vi "BlurredRegistration.vi"(8 "error in":errorcluster, 9 "Gaussian blur parameters":T1={"large sigma"=20.0, "small sigma"=4.0, "equalize?"=FALSE}, 10 "roy":T2, 11 "rob":T2) -> (0 "error out":errorcluster, 1 "alignment quality":dbl, 2 "y displacement":dbl, 3 "x displacement":dbl)   [LabVIEW 2012]
uses:
  <vilib>/vision/Image Controls.llb/IMAQ Image.ctl
  Gaussian blur parameters.ctl
  <vilib>/vision/NI_Vision_Development_Module.lvlib
panel:
  out "gaussian roy":T2(plugin-control)
  out "gaussian rob":T2(plugin-control)
  out "gaussian cc":T2(plugin-control)
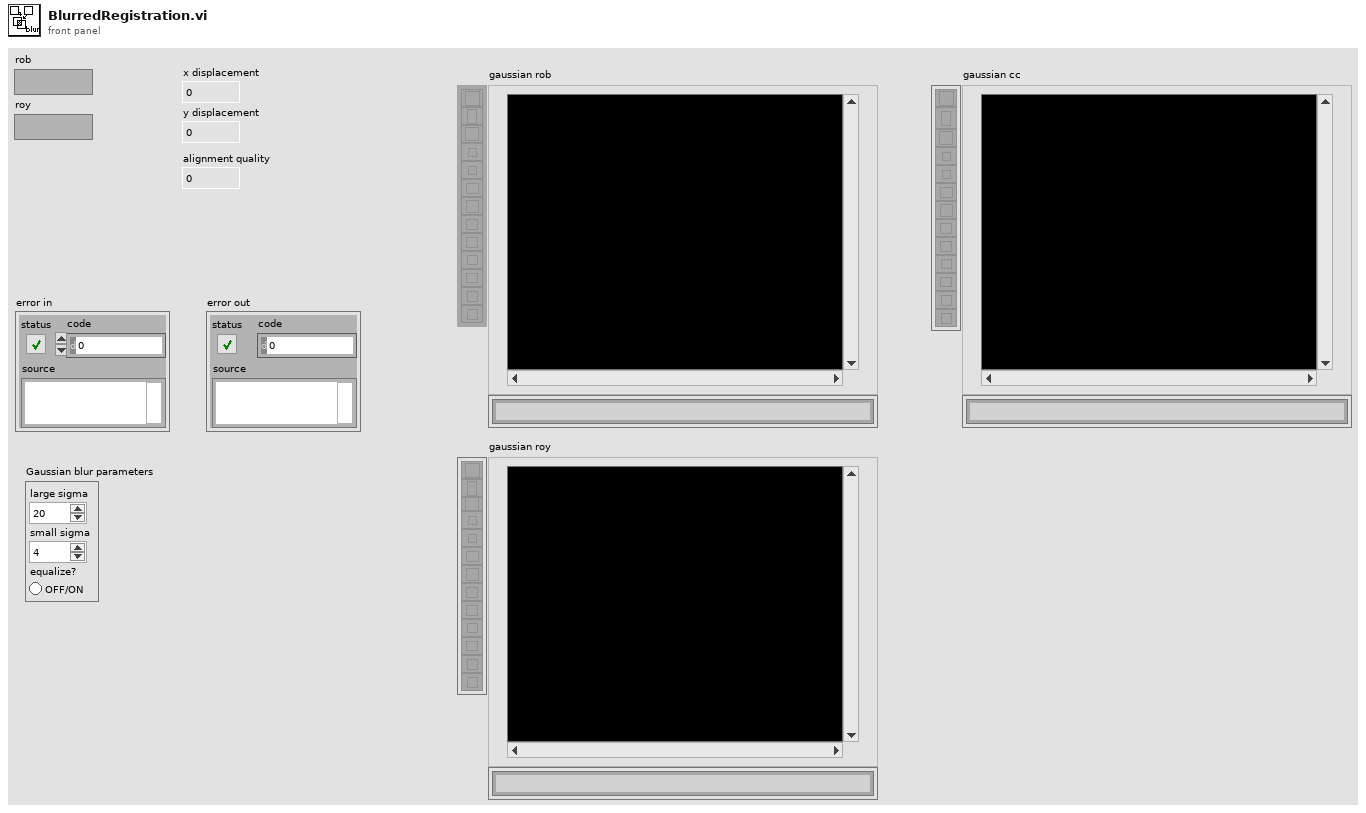
[diagram p1: front panel]
types:
  T1 = typedef "Gaussian blur parameters.ctl" = cluster{"large sigma":sgl, "small sigma":sgl, "equalize?":bool}
  T2 = typedef "IMAQ Image.ctl" = refnum<image>
  T3 = typedef "Image Type" = u32
  T4 = cluster{"histogram":u32[], "Minimal Value":sgl, "Maximal Value":sgl, "Starting Value":sgl, "Interval Width":sgl, "Mean Value":sgl, "Standard  Variation":sgl, "Area (pixels)":i32}
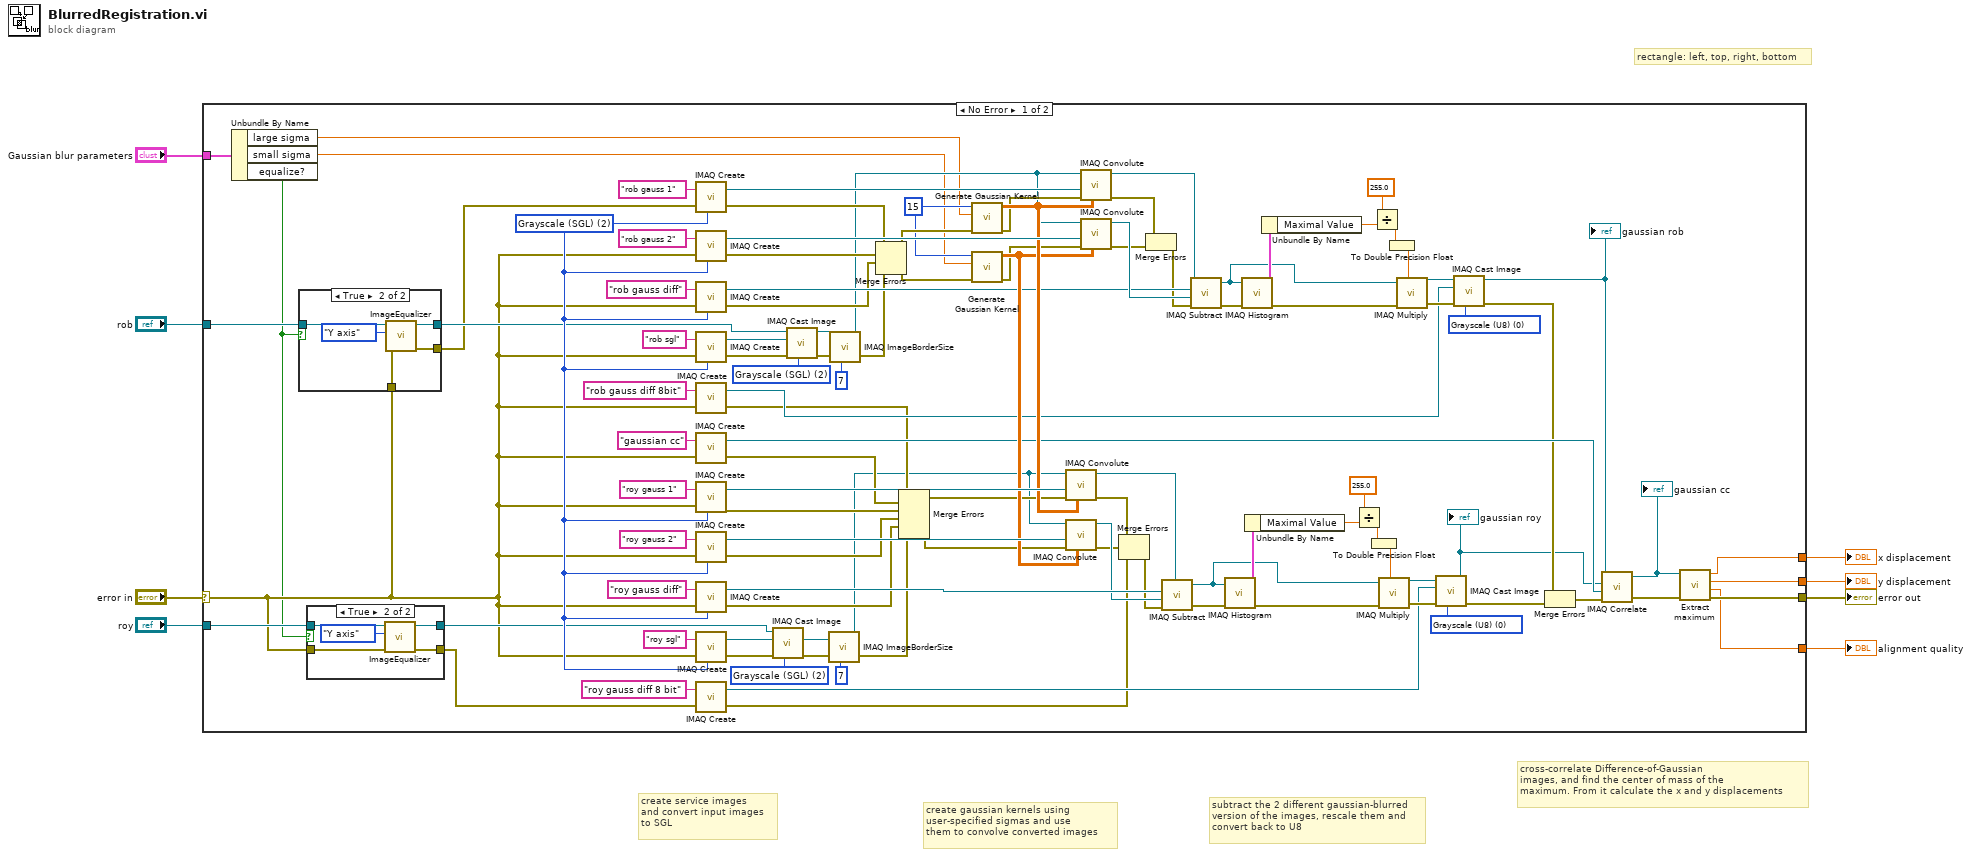
[diagram p0: block diagram]
diagram:
  # "rectangle: left, top, right, bottom"
  # "cross-correlate Difference-of-Gaussian\nimages, and find the center of mass of the \nmaximum. From it calculate the x and y displacements"
  # "subtract the 2 different gaussian-blurred\nversion of the images, rescale them and \nconvert back to U8"
  # "create gaussian kernels using\nuser-specified sigmas and use \nthem to convolve converted images"
  # "create service images\nand convert input images\nto SGL"
  n1 = case shown="No Error" "error in" {
    selector: "error in" -> [w21 w130]
    tunnel: [w17 w130] -> w7
    tunnel: "roy" -> [w23 _]
    tunnel: "rob" -> [w26 _]
    tunnel: [w15 _] -> w3
    tunnel: [w16 _] -> w2
    tunnel: [w14 _] -> w4
    tunnel: "Gaussian blur parameters" -> [w12 _]
    frame No Error {
      w35 = T3 2 items=["Grayscale (U8)", "Grayscale (I16)", "Grayscale (SGL)", "Complex (CSG)", "RGB (U32)", "HSL (U32)", "RGB (U64)", "Grayscale (U16)"] ("Image Type")
      w40 = T3 2 items=["Grayscale (U8)", "Grayscale (I16)", "Grayscale (SGL)", "Complex (CSG)", "RGB (U32)", "HSL (U32)", "RGB (U64)", "Grayscale (U16)"] ("Image Type")
      w55 = T3 0 items=["Grayscale (U8)", "Grayscale (I16)", "Grayscale (SGL)", "Complex (CSG)", "RGB (U32)", "HSL (U32)", "RGB (U64)", "Grayscale (U16)"] ("Image Type")
      w62 = T3 0 items=["Grayscale (U8)", "Grayscale (I16)", "Grayscale (SGL)", "Complex (CSG)", "RGB (U32)", "HSL (U32)", "RGB (U64)", "Grayscale (U16)"] ("Image Type")
      w73 = T3 2 items=["Grayscale (U8)", "Grayscale (I16)", "Grayscale (SGL)", "Complex (CSG)", "RGB (U32)", "HSL (U32)", "RGB (U64)", "Grayscale (U16)"] ("Image Type")
      w76 = 15 ("kernel size (odd number)")
      n2 = Unbundle By Name(w12) -> ("large sigma"=w11:sgl, "small sigma"=w10:sgl, "equalize?"=w9:bool)
      n3 = case shown="True" w9 {
        tunnel: w26 -> [w124 w129]
        tunnel: [w124 w128] -> w25
        tunnel: [w123 w126] -> w24
        tunnel: w21 -> [w123 w125]
        frame False {
        }
        frame True {
          n4 = call "ImageEqualizer.vi"("error in (no error)"=w125, "axis to equalize"=enum16{"X axis", "Y axis"}."Y axis", "Image in"=w129) -> ("error out"=w126:errorcluster, "Image out"=w128:T2)  [unwired: 7 in]
        }
      }
      n5 = case shown="True" w9 {
        tunnel: w23 -> [w117 w121]
        tunnel: [w117 w120] -> w22
        tunnel: w21 -> [w116 w119]
        tunnel: [w116 w118] -> w13
        frame False {
        }
        frame True {
          n6 = call "ImageEqualizer.vi"("error in (no error)"=w119, "axis to equalize"=enum16{"X axis", "Y axis"}."Y axis", "Image in"=w121) -> ("error out"=w118:errorcluster, "Image out"=w120:T2)  [unwired: 7 in]
        }
      }
      n7 = call "IMAQ Create"("Image Name"="rob gauss 1", "Image Type"=w73, "error in (no error)"=w24) -> ("New Image"=w104:T2, "error out"=w92:errorcluster)  [unwired: 2 in]
      n8 = call "IMAQ Create"("Image Name"="rob gauss 2", "Image Type"=w73, "error in (no error)"=w21) -> ("New Image"=w103:T2, "error out"=w91:errorcluster)  [unwired: 2 in]
      n9 = call "IMAQ Create"("Image Name"="rob gauss diff", "Image Type"=w73, "error in (no error)"=w21) -> ("New Image"=w96:T2, "error out"=w90:errorcluster)  [unwired: 2 in]
      n10 = call "IMAQ Create"("Image Name"="rob sgl", "Image Type"=w73, "error in (no error)"=w21) -> ("New Image"=w44:T2, "error out"=w43:errorcluster)  [unwired: 2 in]
      n11 = call "IMAQ Create"("Image Name"="rob gauss diff 8bit", "error in (no error)"=w21) -> ("New Image"=w63:T2, "error out"=w33:errorcluster)  [unwired: 3 in]
      n12 = call "IMAQ Create"("Image Name"="gaussian cc", "error in (no error)"=w21) -> ("New Image"=w70:T2, "error out"=w34:errorcluster)  [unwired: 3 in]
      n13 = call "IMAQ Create"("Image Name"="roy gauss 1", "Image Type"=w73, "error in (no error)"=w21) -> ("New Image"=w102:T2, "error out"=w82:errorcluster)  [unwired: 2 in]
      n14 = call "IMAQ Create"("Image Name"="roy gauss 2", "Image Type"=w73, "error in (no error)"=w21) -> ("New Image"=w101:T2, "error out"=w83:errorcluster)  [unwired: 2 in]
      n15 = call "IMAQ Create"("Image Name"="roy gauss diff", "Image Type"=w73, "error in (no error)"=w21) -> ("New Image"=w95:T2, "error out"=w81:errorcluster)  [unwired: 2 in]
      n16 = call "IMAQ Create"("Image Name"="roy sgl", "Image Type"=w73, "error in (no error)"=w21) -> ("New Image"=w39:T2, "error out"=w37:errorcluster)  [unwired: 2 in]
      n17 = call "IMAQ Create"("Image Name"="roy gauss diff 8 bit", "error in (no error)"=w13) -> ("New Image"=w53:T2, "error out"=w29:errorcluster)  [unwired: 3 in]
      n18 = call "IMAQ Cast Image"("Image Type"=w35, "error in (no error)"=w37, "Image Dst"=w39, "Image Src"=w22) -> ("error out"=w36:errorcluster, "Image Dst Out"=w38:T2)  [unwired: 6 in]
      n19 = call "IMAQ Cast Image"("Image Type"=w40, "error in (no error)"=w43, "Image Dst"=w44, "Image Src"=w25) -> ("error out"=w42:errorcluster, "Image Dst Out"=w41:T2)  [unwired: 6 in]
      n20 = call "IMAQ ImageBorderSize"("Image"=w38, "Image border size in"=7, "error in (no error)"=w36) -> ("Image Out"=w30:T2, "error out"=w31:errorcluster)  [unwired: 1 in, 1 out]
      n21 = call "IMAQ ImageBorderSize"("Image"=w41, "Image border size in"=7, "error in (no error)"=w42) -> ("Image Out"=w72:T2, "error out"=w32:errorcluster)  [unwired: 1 in, 1 out]
      n22 = Merge Errors(w92, w91, w90, w32) -> (w89:errorcluster)
      n23 = Merge Errors(w33, w34, w82, w83, w81, w31) -> (w80:errorcluster)
      n24 = call "Generate Gaussian Kernel.vi"("error in (no error)"=w89, "sigma"=w11, "kernel size (odd number)"=w76) -> ("error out"=w88:errorcluster, "Kernel"=w100:sgl[][])  [unwired: 7 in]
      n25 = call "Generate Gaussian Kernel.vi"("error in (no error)"=w89, "sigma"=w10, "kernel size (odd number)"=w76) -> ("error out"=w87:errorcluster, "Kernel"=w99:sgl[][])  [unwired: 7 in]
      n26 = call "IMAQ Convolute"("Kernel"=w100, "error in (no error)"=w80, "Image Dst"=w102, "Image Src"=w30) -> ("error out"=w78:errorcluster, "Image Dst Out"=w94:T2)  [unwired: 6 in]
      n27 = call "IMAQ Convolute"("Kernel"=w99, "error in (no error)"=w80, "Image Dst"=w101, "Image Src"=w30) -> ("error out"=w79:errorcluster, "Image Dst Out"=w93:T2)  [unwired: 6 in]
      n28 = call "IMAQ Convolute"("Kernel"=w100, "error in (no error)"=w88, "Image Dst"=w104, "Image Src"=w72) -> ("error out"=w85:errorcluster, "Image Dst Out"=w98:T2)  [unwired: 6 in]
      n29 = call "IMAQ Convolute"("Kernel"=w99, "error in (no error)"=w87, "Image Dst"=w103, "Image Src"=w72) -> ("error out"=w86:errorcluster, "Image Dst Out"=w97:T2)  [unwired: 6 in]
      n30 = Merge Errors(w78, w79, w29) -> (w77:errorcluster)
      n31 = Merge Errors(w85, w86) -> (w84:errorcluster)
      n32 = call "IMAQ Subtract"("Image Src A"=w94, "Image Dst"=w95, "Image Src B"=w93, "error in (no error)"=w77) -> ("Image Dst Out"=w47:T2, "error out"=w54:errorcluster)  [unwired: 3 in]
      n33 = call "IMAQ Subtract"("Image Src A"=w98, "Image Dst"=w96, "Image Src B"=w97, "error in (no error)"=w84) -> ("Image Dst Out"=w50:T2, "error out"=w71:errorcluster)  [unwired: 3 in]
      n34 = call "IMAQ Histogram"("error in (no error)"=w54, "Image"=w47) -> ("error out"=w46:errorcluster, "Histogram Report"=w61:T4)  [unwired: 8 in]
      n35 = call "IMAQ Histogram"("error in (no error)"=w71, "Image"=w50) -> ("error out"=w49:errorcluster, "Histogram Report"=w69:T4)  [unwired: 8 in]
      n36 = Unbundle By Name(w61) -> ("Maximal Value"=w45:sgl)
      n37 = Unbundle By Name(w69) -> ("Maximal Value"=w48:sgl)
      n38 = Divide(x=sgl 255.0, y=w45) -> (x/y=w59:sgl)
      n39 = To Double Precision Float(number=w59) -> (double precision float=w58:dbl)
      n40 = Divide(x=sgl 255.0, y=w48) -> (x/y=w67:sgl)
      n41 = call "IMAQ Multiply"("Image Src A"=w47, "Constant"=w58, "error in (no error)"=w46) -> ("Image Dst Out"=w56:T2, "error out"=w57:errorcluster)  [unwired: 4 in]
      n42 = To Double Precision Float(number=w67) -> (double precision float=w66:dbl)
      n43 = call "IMAQ Multiply"("Image Src A"=w50, "Constant"=w66, "error in (no error)"=w49) -> ("Image Dst Out"=w64:T2, "error out"=w65:errorcluster)  [unwired: 4 in]
      n44 = call "IMAQ Cast Image"("Image Type"=w55, "error in (no error)"=w57, "Image Dst"=w53, "Image Src"=w56) -> ("error out"=w52:errorcluster, "Image Dst Out"=w28:T2)  [unwired: 6 in]
      "gaussian roy" <- w28
      n45 = call "IMAQ Cast Image"("Image Type"=w62, "error in (no error)"=w65, "Image Dst"=w63, "Image Src"=w64) -> ("error out"=w51:errorcluster, "Image Dst Out"=w27:T2)  [unwired: 6 in]
      "gaussian rob" <- w27
      n46 = Merge Errors(w51, w52) -> (w20:errorcluster)
      n47 = call "IMAQ Correlate"("Image Src"=w27, "Image Template"=w28, "Image Dst"=w70, "error in (no error)"=w20) -> ("Image Dst Out"=w18:T2, "error out"=w19:errorcluster)  [unwired: 3 in]
      "gaussian cc" <- w18
      n48 = call "Extract maximum.vi"("error in (no error)"=w19, "Image in"=w18) -> ("error out"=w17:errorcluster, "Max value"=w14:dbl, "y translation"=w15:dbl, "x translation"=w16:dbl)  [unwired: 6 in]
    }
    frame Error {
    }
  }
  "error out" <- w7
  "x displacement" <- w2
  "y displacement" <- w3
  "alignment quality" <- w4
